vi "TranferNormal.vi"(2 "error in (no error)":errorcluster) -> (0 "error out":errorcluster)   [LabVIEW 2009]
doc: "Set transfer swicth to normal"
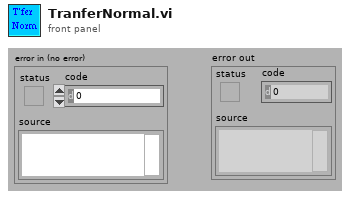
[diagram p1: front panel]
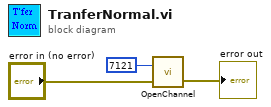
[diagram p0: block diagram]
diagram:
  n1 = call "OpenChannel.vi"("error in (no error)"="error in (no error)", "Channel ID"=7121) -> ("error out"=→"error out":errorcluster)  [unwired: 1 in]
